vi "Init.vi"(8 "error in (no error)":errorcluster, 11 "Input Name":string) -> (0 "error out":errorcluster, 3 "GetInputVolume out":refnum<class "GetInputVolume.lvclass">)   [LabVIEW 2020, in "obs-websocket.lvlib" / "GetInputVolume.lvclass"]
uses:
  GetInputVolume.lvclass
  GetInputVolume.lvclass/GetInputVolume.ctl
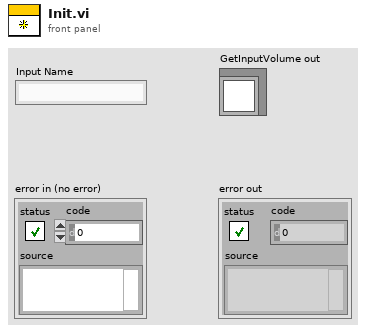
[diagram p1: front panel]
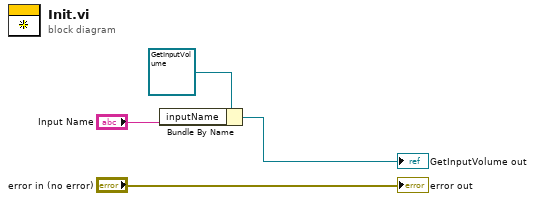
[diagram p0: block diagram]
diagram:
  n1 = Bundle By Name(cluster=refnum<class "GetInputVolume.lvclass"> refnum ("GetInputVolume in"), "inputName"="Input Name") -> (→"GetInputVolume out":refnum<class "GetInputVolume.lvclass">)
  "error out" <- "error in (no error)"
